vi "Parse Alarm Error.vi"(0 "errors":bool[][](array[boolean]), 5 "error description":string[](array[string])) -> (4 "error description":string, 8 "error":bool)   [LabVIEW 2019]
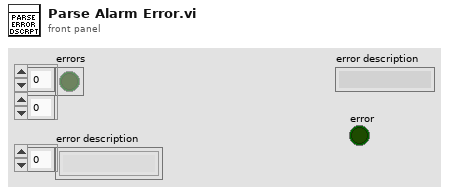
[diagram p1: front panel]
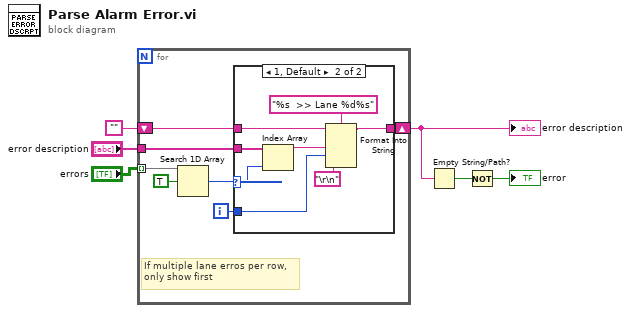
[diagram p0: block diagram]
diagram:
  n1 = for {
    tunnel: "errors" -> [w13] mode=indexing
    shift-right: [w9] -> w3
    shift-left: "" -> [w10]
    tunnel: "error description" -> [w8]
    i -> [w7]
    # "If multiple lane erros per row,\nonly show first"
    n2 = Search 1D Array(1D array=w13, element=TRUE) -> (index of element=w11:i32)  [unwired: 1 in]
    n3 = case shown="1, Default" w11 {
      selector: w11 -> [_ w18]
      tunnel: w10 -> [w14 w22]
      tunnel: [w14 w21] -> w9
      tunnel: w8 -> [_ w19]
      tunnel: w7 -> [_ w17]
      frame -1 {
      }
      frame 1, Default {
        n4 = Index Array(array=w19, index=w18) -> (element=w15:string)
        n5 = Format Into String(format string="%s  >> Lane %d%s", initial string=w22, w15, w17, "\r\n") -> (resulting string=w21:string)  [unwired: 1 in, 1 out]
      }
    }
  }
  "error description" <- w3
  n6 = Empty String/Path?(string/path=w3) -> (empty?=w2:bool)
  n7 = Not(x=w2) -> (.not. x?=→"error":bool)
